vi "generate object.vi"(10 "json string values":string[](array[string]), 11 "json string keys":string[](array[string])) -> (3 "object string":string)   [LabVIEW 2013, in "json generator.lvlib"]
uses:
  json generator.lvlib
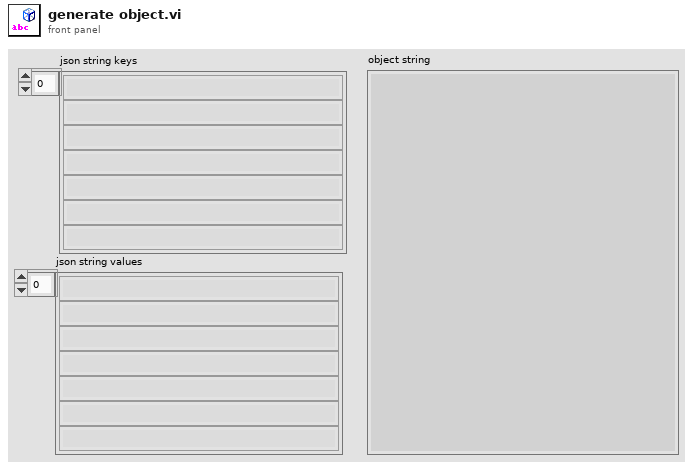
[diagram p1: front panel]
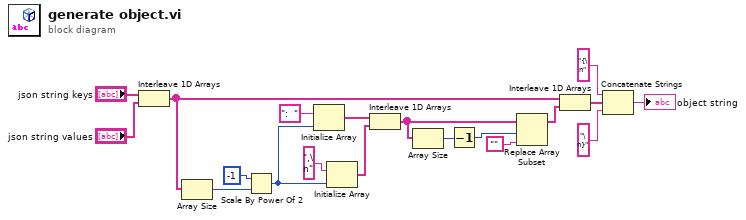
[diagram p0: block diagram]
diagram:
  n1 = Interleave 1D Arrays("json string keys", "json string values") -> (w2:string[])
  n2 = Array Size(array=w2) -> (size(s)=w7:i32)
  n3 = Scale By Power Of 2(n=i16 -1, x=w7) -> (x*2^n=w11:i32)
  n4 = Initialize Array(":  ", w11) -> (w9:string[])
  n5 = Initialize Array(",\n", w11) -> (w10:string[])
  n6 = Interleave 1D Arrays(w9, w10) -> (w6:string[])
  n7 = Array Size(array=w6) -> (size(s)=w5:i32)
  n8 = Decrement(x=w5) -> (x-1=w4:i32)
  n9 = Replace Array Subset(array=w6, new element="", index=w4) -> (w3:string[])
  n10 = Interleave 1D Arrays(w2, w3) -> (w1:string[])
  n11 = Concatenate Strings("{\n" ("string"), w1, "\n}" ("string")) -> (→"object string":string)
